vi "Save-to-file-by-value.vi"(8 "error in (no error)":errorcluster, 10 "Values to save":T2, 11 "Reference in":T1) -> (0 "error out":errorcluster, 3 "Reference out":T1)   [LabVIEW 2013, in "SettingsFile.lvlib" / "SettingsFile.lvclass"]
uses:
  SettingsFile.lvclass
  Object-reference.ctl
  Values-to-save.ctl
  Messages.ctl
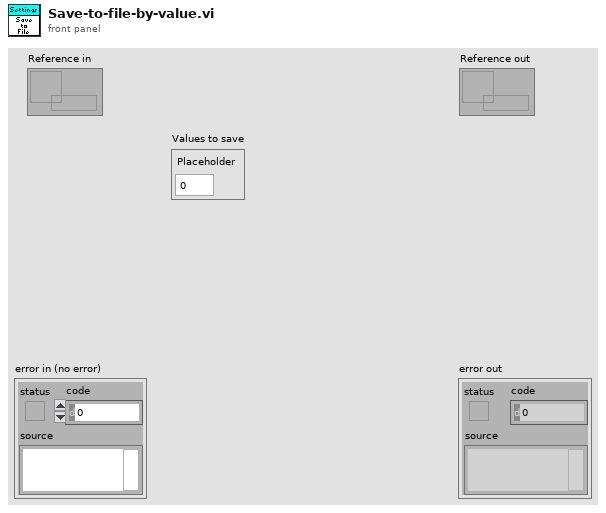
[diagram p1: front panel]
types:
  T1 = typedef "SettingsFile.lvlib/SettingsFile.lvclass/Object-reference.ctl" = refnum<data-value>
  T2 = typedef "SettingsFile.lvlib/SettingsFile.lvclass/Values-to-save.ctl" = cluster{"Placeholder":dbl}
  T3 = typedef "SettingsFile.lvlib/SettingsFile.lvclass/Messages.ctl" = enum16{"Time out", "User cancel", "Module cancel", "File format change"}
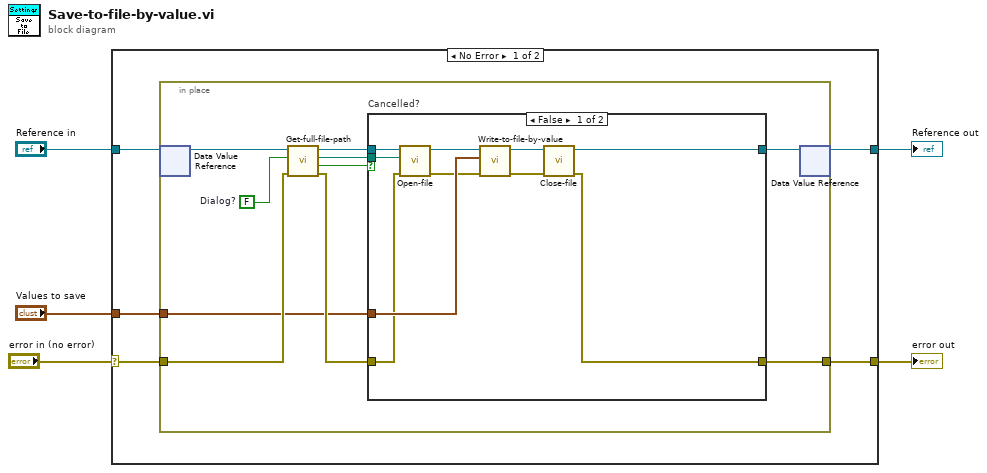
[diagram p0: block diagram]
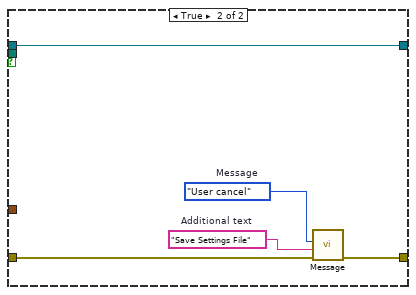
[diagram p2: hidden frame]
diagram:
  n1 = case shown="No Error" "error in (no error)" {
    selector: "error in (no error)" -> [w8 w37]
    tunnel: [w7 w37] -> w4
    tunnel: "Values to save" -> [w6 _]
    tunnel: "Reference in" -> [w10 w36]
    tunnel: [w9 w36] -> w1
    frame No Error {
      n2 = in-place {
        in-place-border: w8 -> [w15]
        in-place-border: [w13] -> w7
        in-place-border: w6 -> [w12]
        w19 = FALSE  # Dialog?
        n3 = in-place-dvr #1(w10) -> (w20:refnum<class "SettingsFile.lvclass">)  [unwired: 1 out]
        n4 = call "Get-full-file-path.vi"("error in (no error)"=w15, "Dialog?"=w19, "SettingsFile in"=w20) -> ("error out"=w14:errorcluster, "Cancelled?"=w18:bool, "Full path"=w17:path, "SettingsFile out"=w16:refnum<class "SettingsFile.lvclass">)  [unwired: 5 in]
        n5 = case "Cancelled?" shown="False" w18 {
          tunnel: w17 -> [w29 _]
          tunnel: w16 -> [w30 w31]
          tunnel: w14 -> [w23 w35]
          tunnel: [w22 w34] -> w13
          tunnel: w12 -> [w27 _]
          tunnel: [w21 w31] -> w11
          frame False {
            n6 = call "Open-file.vi"("error in (no error)"=w23, "Full path"=w29, "SettingsFile in"=w30) -> ("error out"=w26:errorcluster, "SettingsFile out"=w28:refnum<class "SettingsFile.lvclass">)  [unwired: 6 in, 1 out]
            n7 = call "Write-to-file-by-value.vi"("error in (no error)"=w26, "Values to save"=w27, "SettingsFile in"=w28) -> ("error out"=w24:errorcluster, "SettingsFile out"=w25:refnum<class "SettingsFile.lvclass">)  [unwired: 7 in]
            n8 = call "Close-file.vi"("error in (no error)"=w24, "SettingsFile in"=w25) -> ("error out"=w22:errorcluster, "SettingsFile out"=w21:refnum<class "SettingsFile.lvclass">)  [unwired: 8 in]
          }
          frame True {
            w32 = Messages."User cancel"  # Message
            w33 = "Save Settings File"  # Additional text
            n9 = call "Message.vi"("error in (no error)"=w35, "Additional text"=w33, "Message"=w32) -> ("error out"=w34:errorcluster)  [unwired: 8 in]
          }
        }
        n10 = in-place-dvr #1(w11) -> (w9:T1)  [unwired: 1 out]
      }
    }
    frame Error {
    }
  }
  "error out" <- w4
  "Reference out" <- w1
